vi "FdxCmdTxControlCvi.vi"(8 "error in":errorcluster, 9 "TxControl":T1 {"ExtendedStopMode" items=["FDX_ESTOP_NOT_USED", "FDX_ESTOP_EXT_TRG", "FDX_ESTOP_EXT_TRG_RESTART", "FDX_ESTOP_TIME"]; "StartMode" items=["FDX_STOP", "FDX_START", "FDX_START_TRG", "FDX_START_TIME"]}, 11 "InstrumentHandle_port in":u32) -> (0 "error out":errorcluster, 3 "InstrumentHandle_port out":u32)   [LabVIEW 2020, in "AIM664LV.lvlib"]
doc: "This function is used to control the transmit operation of the board."
uses:
  AIM664LV.lvlib
  AFDX_LibraryAdmin/FdxGlobalDllPath.vi
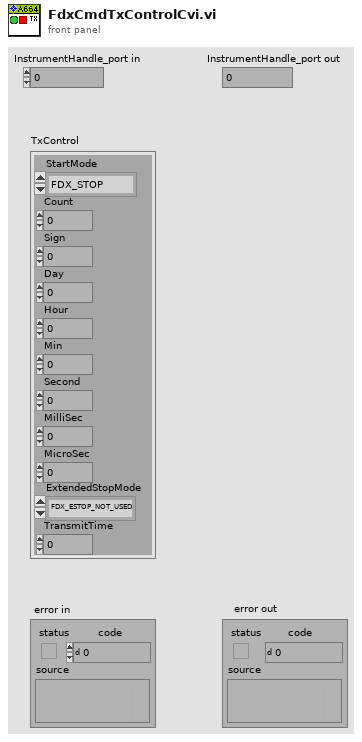
[diagram p1: front panel]
types:
  T1 = cluster{"StartMode":i32, "Count":u32, "Sign":i32, "Day":u32, "Hour":u32, "Min":u32, "Second":u32, "MilliSec":u32, "MicroSec":u32, "ExtendedStopMode":i32, "TransmitTime":u32}
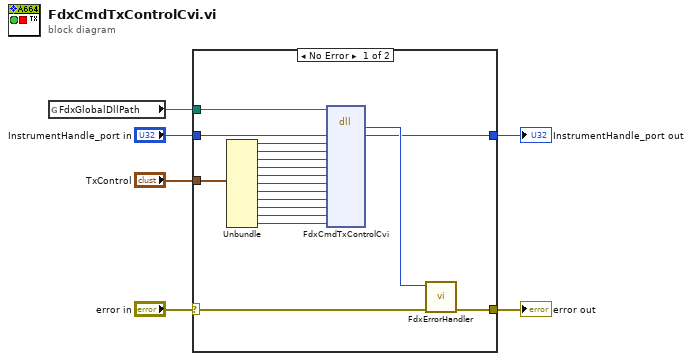
[diagram p0: block diagram]
diagram:
  n1 = global read "FdxGlobalDllPath.vi" "FdxGlobalDllPath"() -> (w4:path)
  n2 = case shown="No Error" "error in" {
    selector: "error in" -> [w23 w26]
    tunnel: [w24 w26] -> w6
    tunnel: w4 -> [w10 _]
    tunnel: [w9 w25] -> w3
    tunnel: "InstrumentHandle_port in" -> [w8 w25]
    tunnel: "TxControl" -> [w7 _]
    frame No Error {
      n3 = Unbundle(w7) -> ("StartMode"=w21:i32, "Count"=w20:u32, "Sign"=w19:i32, "Day"=w18:u32, "Hour"=w17:u32, "Min"=w16:u32, "Second"=w15:u32, "MilliSec"=w14:u32, "MicroSec"=w13:u32, "ExtendedStopMode"=w12:i32, "TransmitTime"=w11:u32)
      n4 = dll-call lib="aim_fdx.19.dll" fn="FdxCmdTxControlCvi"(path in=w10, "InstrumentHandle"=w8, "StartMode"=w21, "Count"=w20, "Sign"=w19, "Day"=w18, "Hour"=w17, "Min"=w16, "Second"=w15, "MilliSec"=w14, "MicroSec"=w13, "ExtendedStopMode"=w12, "TransmitTime"=w11) -> ("status"=w22:i32, "InstrumentHandle"=w9:u32)  [unwired: 13 in, 2 out]
      n5 = call "FdxErrorHandler.vi"("error in"=w23, "AIM Error"=w22) -> ("error out"=w24:errorcluster)  [unwired: 9 in]
    }
    frame Error {
    }
  }
  "error out" <- w6
  "InstrumentHandle_port out" <- w3
